vi "Switch Relays.vi"(8 "error in":errorcluster, 10 "Alias":string="DUT0", 11 "RelayMode":T1) -> (0 "error out":errorcluster={"status"=TRUE, "code"=-200099, "source"="DAQmx Create Channel (DO-Digital Output).vi:6970001<append>\n<B>Task Name: </B>_unnamedTask<1>"})   [LabVIEW 2021]
uses:
  Controls/Relay States.ctl
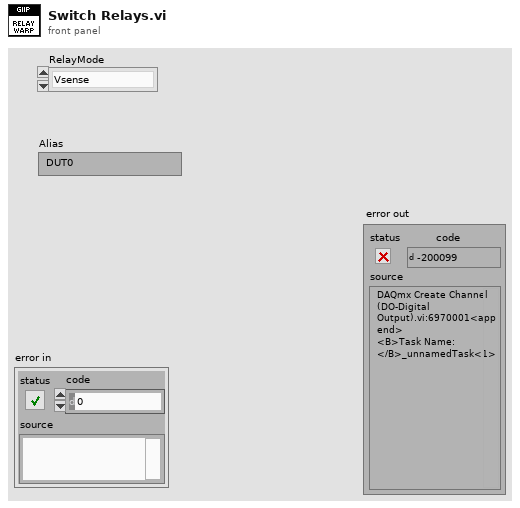
[diagram p1: front panel]
types:
  T1 = typedef "Relay States.ctl" = enum16{"Vsense", "Thermistor", "ACIR", "HiPOT1", "HiPOT2"}
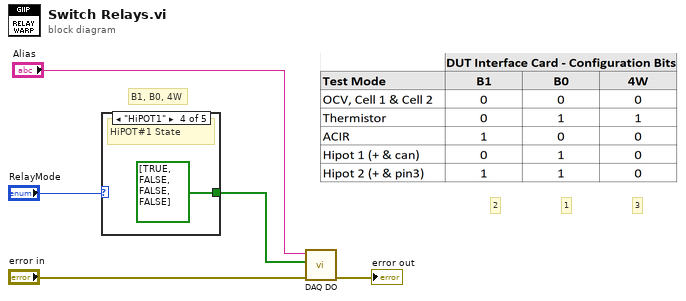
[diagram p0: block diagram]
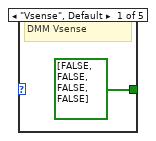
[diagram p2: hidden frame]
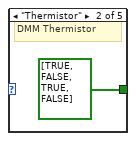
[diagram p3: hidden frame]
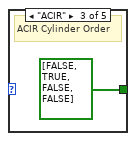
[diagram p4: hidden frame]
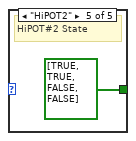
[diagram p5: hidden frame]
diagram:
  # "3"
  # "2"
  # "1"
  # "B1, B0, 4W"
  n1 = case shown="\"HiPOT1\"" "RelayMode" {
    tunnel: [bool[] [FALSE, FALSE, FALSE, FALSE] bool[] [TRUE, FALSE, TRUE, FALSE] bool[] [FALSE, TRUE, FALSE, FALSE] bool[] [TRUE, FALSE, FALSE, FALSE] bool[] [TRUE, TRUE, FALSE, FALSE]] -> w1
    frame "Vsense", Default {
      # "DMM Vsense"
    }
    frame "Thermistor" {
      # "DMM Thermistor"
    }
    frame "ACIR" {
      # "ACIR Cylinder Order"
    }
    frame "HiPOT1" {
      # "HiPOT#1 State"
    }
    frame "HiPOT2" {
      # "HiPOT#2 State"
    }
  }
  n2 = call "DAQ DO.vi"("error in"="error in", "Relay Mode"=w1, "Alias"="Alias") -> ("error out"=→"error out":errorcluster)  [unwired: 8 in]
